vi "UDP__Send.vi"(4 "Remote Port":u16, 5 "Local Port":u16, 6 "Remote MAC Address (hex)":string="\u0000\u0000\u0000\u0000\u0000\u0000", 7 "Local MAC Address (hex)":string="\u0000\u0000\u0000\u0000\u0000\u0000", 8 "error in":errorcluster, 10 "Command and Data":string, 11 "UDP Network Connection in":refnum<k16>) -> (0 "error out":errorcluster, 3 "UDP Network Connection out":refnum<k16>)   [LabVIEW 2014, in "hse-network.lvlib"]
doc: "____\nHAMPEL SOFTWARE ENGINEERING v0.7.0 (2018-07-16 18:12)"
uses:
  hse-network.lvlib
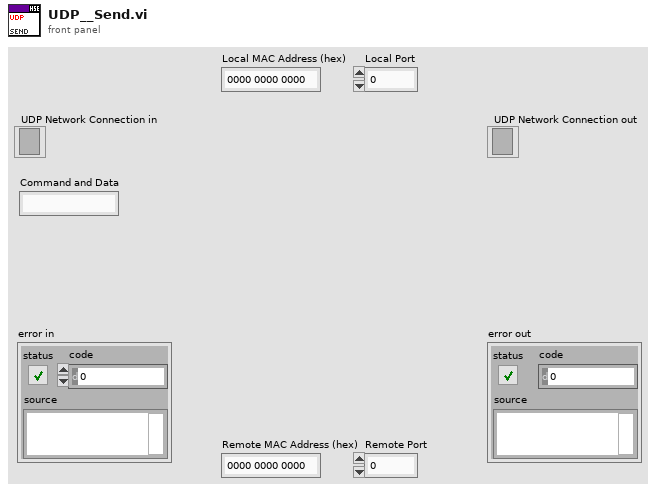
[diagram p1: front panel]
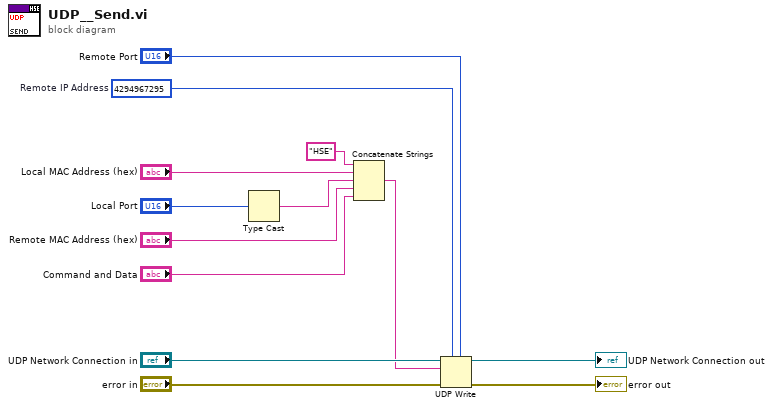
[diagram p0: block diagram]
diagram:
  w8 = u32 4294967295  # Remote IP Address
  n1 = Type Cast(x="Local Port") -> (*(type *) &x=w1:string)  [unwired: 1 in]
  n2 = Concatenate Strings("HSE" ("format string"), "Local MAC Address (hex)", w1, "Remote MAC Address (hex)", "Command and Data") -> (w7:string)
  n3 = UDP Write(address=w8, port or service name="Remote Port", connection ID="UDP Network Connection in", data in=w7, 8:"error in") -> (error out=→"error out":errorcluster, 3:→"UDP Network Connection out":refnum<k16>)  [unwired: 1 out]
